vi "Configure ALL AI DAQ Settings.vi"(1 "AI TaskNames":string[](array[string]), 5 "DAQNode Dict":T1, 11 "error in (no error)":errorcluster, 14 "Simulate":bool) -> (6 "DAQNode Dict out":T1, 15 "error out":errorcluster)   [LabVIEW 2022 SP3, in "DAQ.lvclass"]
doc: "Developed by Kevin Thompson\nkevin@thompsonengineering.net\n\nCopyright 2018-2020\nThompson Engineering, LLC"
uses:
  DAQ.lvclass
  <vilib>/TELLC/Dynamic CVT API/TD Dynamic CVT DVR--ref.ctl
  DataTypes/TD AI TaskIO.ctl
  DataTypes/TD AI Instrument Settings--cluster.ctl
  DataTypes/TD AI InstSettings--cluster.ctl
  Process/ProcessSupport/TD SimAI Ranges--cluster.ctl
  <vilib>/DAQmx/configure/timing.llb/DAQmx Timing (Sample Clock).vi
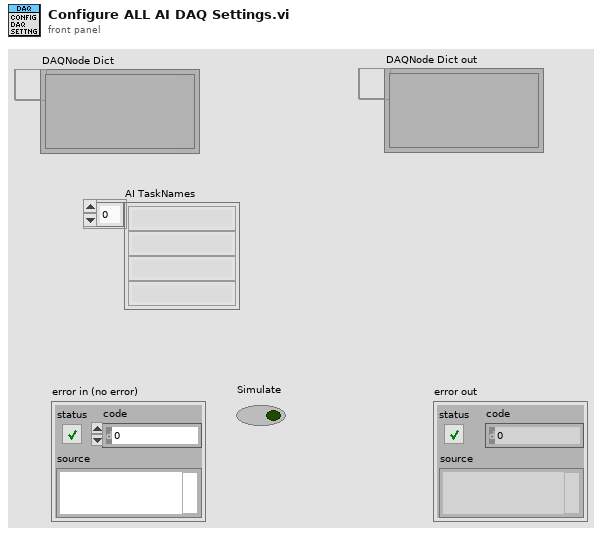
[diagram p1: front panel]
types:
  T1 = typedef "TD Dynamic CVT DVR--ref.ctl" = refnum<data-value>
  T2 = typedef "DAQ.lvclass/TD AI Instrument Settings--cluster.ctl" = cluster{"Disable":bool, "AI TaskName":string, "AI InstSettings":T3, "SimAI Ranges":T4}
  T3 = typedef "DAQ.lvclass/TD AI InstSettings--cluster.ctl" = cluster{"DaqRate":dbl, "NumSamples":i32}
  T4 = typedef "DAQ.lvclass/TD SimAI Ranges--cluster.ctl" = cluster{"lo":dbl, "hi":dbl}
  T5 = typedef "DAQ.lvclass/TD AI TaskIO.ctl" = cluster{"AI TaskName":string, "IONames":string[], "DAQmx AI TaskRef":refnum<k21>}
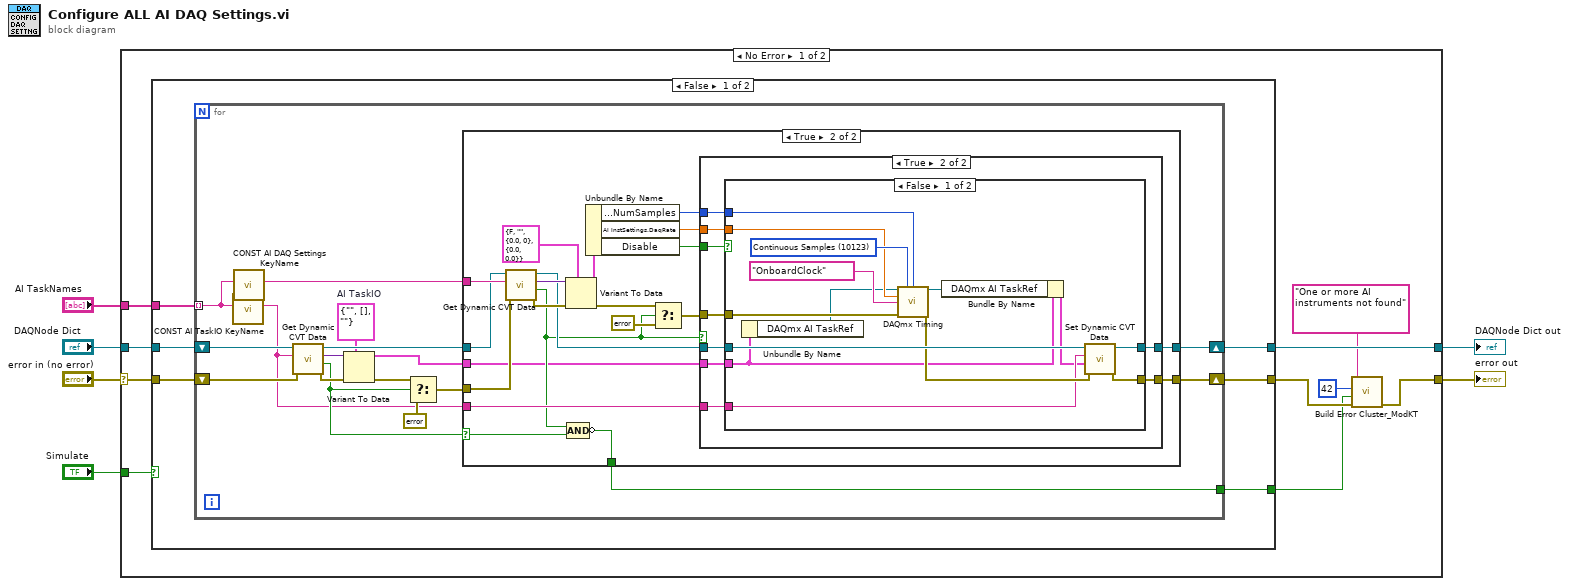
[diagram p0: block diagram]
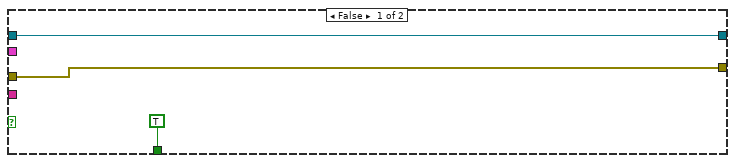
[diagram p2: hidden frame]
diagram:
  n1 = case shown="No Error" "error in (no error)" {
    selector: "error in (no error)" -> [w13 w94]
    tunnel: "DAQNode Dict" -> [w16 w93]
    tunnel: "AI TaskNames" -> [w15 _]
    tunnel: [w11 w94] -> w4
    tunnel: [w14 w93] -> w3
    tunnel: "Simulate" -> [w12 _]
    frame No Error {
      n2 = case shown="False" w12 {
        tunnel: w16 -> [w22 w91]
        tunnel: w15 -> [w17 _]
        tunnel: w13 -> [w21 w92]
        tunnel: [w20 w92] -> w10
        tunnel: [w19 w91] -> w14
        tunnel: [w18 _] -> w7
        frame False {
          n3 = for {
            tunnel: [w26] -> w18
            shift-right: [w36] -> w19
            shift-left: w22 -> [w39]
            shift-right: [w37] -> w20
            shift-left: w21 -> [w38]
            tunnel: w17 -> [w24] mode=indexing
            w23 = T5 {"AI TaskName"="", "IONames"=[], "DAQmx AI TaskRef"=""}  # AI TaskIO
            n4 = call "CONST AI TaskIO KeyName.vi"("AI TaskName"=w24) -> ("AI TaskIO (KeyName)"=w25:string)  [unwired: 10 in]
            n5 = call "CONST AI DAQ Settings KeyName.vi"("AI TaskName"=w24) -> ("AI DAQ Settings (KeyName)"=w33:string)  [unwired: 10 in]
            n6 = call <vilib>:"Get Dynamic CVT Data.vi"("error in (no error)"=w38, "DataName"=w25, "dCVT DVR"=w39) -> ("error out"=w35:errorcluster, "found"=w27:bool, "value"=w34:variant, "dCVT DVR out"=w32:T1)  [unwired: 5 in]
            n7 = Variant To Data(error in=w35, type=w23, Variant=w34) -> (data=w30:T5, error out=w29:errorcluster)
            n8 = Select(t=w29, s=w27, f=errorcluster {"status"=FALSE, "code"=0, "source"=""} ("error constant")) -> (s? t:f=w31:errorcluster)
            n9 = case shown="True" w27 {
              selector: w27 -> [_ w46]
              tunnel: [w41 w63] -> w36
              tunnel: [w42 w62] -> w37
              tunnel: w33 -> [_ w59]
              tunnel: w32 -> [w41 w58]
              tunnel: w31 -> [w42 w56]
              tunnel: w30 -> [_ w43]
              tunnel: w25 -> [_ w49]
              tunnel: [TRUE w44] -> w26
              frame False {
              }
              frame True {
                n10 = call <vilib>:"Get Dynamic CVT Data.vi"("error in (no error)"=w56, "DataName"=w59, "dCVT DVR"=w58) -> ("error out"=w60:errorcluster, "found"=w45:bool, "value"=w61:variant, "dCVT DVR out"=w57:T1)  [unwired: 5 in]
                n11 = Variant To Data(error in=w60, type=T2 {"Disable"=FALSE, "AI TaskName"="", "AI InstSettings"={"DaqRate"=0.0, "NumSamples"=0}, "SimAI Ranges"={"lo"=0.0, "hi"=0.0}} ("AI Settings"), Variant=w61) -> (data=w53:T2, error out=w48:errorcluster)
                n12 = Compound Arithmetic op=AND(w45, w46) -> (invert w44:bool)
                n13 = Unbundle By Name(w53) -> ("AI InstSettings.NumSamples"=w52:i32, "AI InstSettings.DaqRate"=w51:dbl, "Disable"=w50:bool)
                n14 = Select(t=w48, s=w45, f=errorcluster {"status"=FALSE, "code"=0, "source"=""} ("error constant")) -> (s? t:f=w55:errorcluster)
                n15 = case shown="True" w45 {
                  tunnel: [w65 w74] -> w63
                  tunnel: [w64 w73] -> w62
                  tunnel: w57 -> [w65 w72]
                  tunnel: w55 -> [w64 w71]
                  tunnel: w52 -> [_ w70]
                  tunnel: w51 -> [_ w69]
                  tunnel: w50 -> [_ w68]
                  tunnel: w49 -> [_ w67]
                  tunnel: w43 -> [_ w66]
                  frame False {
                  }
                  frame True {
                    n16 = case shown="False" w68 {
                      tunnel: [w88 w89] -> w74
                      tunnel: [w87 w90] -> w73
                      tunnel: w72 -> [w86 w89]
                      tunnel: w71 -> [w84 w90]
                      tunnel: w70 -> [w82 _]
                      tunnel: w69 -> [w81 _]
                      tunnel: w67 -> [w79 _]
                      tunnel: w66 -> [w76 _]
                      frame False {
                        w83 = 10123 items=["Finite Samples"=10178, "Continuous Samples"=10123, "Hardware Timed Single Point"=12522] ("sample mode")
                        n17 = Unbundle By Name(w76) -> ("DAQmx AI TaskRef"=w75:refnum<k21>)
                        n18 = call-poly <vilib>:"DAQmx Timing.vi"("task/channels in"=w75, "sample mode"=w83, "samples per channel"=w82, "rate"=w81, "source"=tag "OnboardClock" ("Sample Clock Source"), "error in"=w84) -> ("task out"=w78:refnum<k21>, "error out"=w85:errorcluster)  [unwired: 8 in]
                        n19 = Bundle By Name(cluster=w76, "DAQmx AI TaskRef"=w78) -> (w77:T5)
                        n20 = call <vilib>:"Set Dynamic CVT Data.vi"("error in (no error)"=w85, "value"=w77, "DataName"=w79, "dCVT DVR"=w86) -> ("error out"=w87:errorcluster, "dCVT DVR out"=w88:T1)  [unwired: 5 in, 1 out]
                      }
                      frame True {
                      }
                    }
                  }
                }
              }
            }
          }
        }
        frame True {
        }
      }
      n21 = call <vilib>:"Build Error Cluster_ModKT .vi"("Prepend String (\"\")"="One or more AI instruments not found" ("Prepend String (\"\")"), "code"=42, "error? (F)"=w7, "error in (no error)"=w10) -> ("error out"=w11:errorcluster)  [unwired: 3 in, 1 out]
    }
    frame Error {
    }
  }
  "error out" <- w4
  "DAQNode Dict out" <- w3
